vi "Demo.vi"() -> ()   [LabVIEW 2018]
panel:
  out "Filtered Signal":dynamicdata(graph)
  out "data":dynamicdata(graph)
  in  "stop (F)":bool
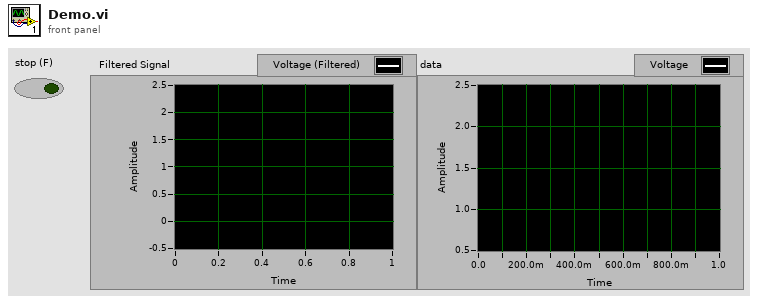
[diagram p1: front panel]
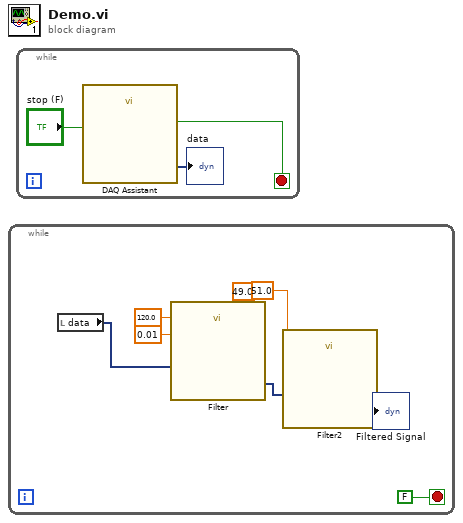
[diagram p0: block diagram]
diagram:
  n1 = while {
    stop <- FALSE stop-if-true
    (unwired) 49.0 ("Lower Cut-Off")
    n2 = local read "data"() -> (w4:dynamicdata)
    n3 = call "Filter"("Lower Cut-Off"=0.01, "Upper Cut-Off"=120.0, "Signal"=w4) -> ("Filtered Signal"=w5:dynamicdata)  [unwired: 7 in, 1 out]
    n4 = call "Filter2"("Lower Cut-Off"=51.0, "Signal"=w5) -> ("Filtered Signal"=→"Filtered Signal":dynamicdata)  [unwired: 8 in, 1 out]
  }
  n5 = while {
    stop <- w9 stop-if-true
    n6 = call "DAQ Assistant"("stop (F)"="stop (F)") -> ("data"=→"data":dynamicdata, "stopped"=w9:bool)  [unwired: 15 in, 2 out]
  }
